vi "DAC Run.vi"(8 "error in":errorcluster, 11 "DAC CS Humid in":refnum<class "DAC CS Humid.lvclass">) -> (0 "error out":errorcluster, 3 "DAC CS Humid out":refnum<class "DAC CS Humid.lvclass">)   [LabVIEW 2019, in "DAC.lvlib" / "DAC CS Humid.lvclass"]
uses:
  DAC CS Humid.lvclass
  C:/Users/wg/Documents/LV_Projects/test-stand/App/DAC/DAC.lvclass
  DAC.lvclass/DAC.ctl
  Results/Results Method.ctl
  Results/DeepU Results/DeepU Results.lvclass
  DAC CS Humid.lvclass/DAC CS Humid.ctl
  <vilib>/DAQmx/miscellaneous.llb/DAQmx Fill In Error Info.vi
  DAC.lvclass
  Results/Results.lvlib
  <vilib>/DAQmx/read.llb/DAQmx Read (Analog 1D Wfm NChan 1Samp).vi
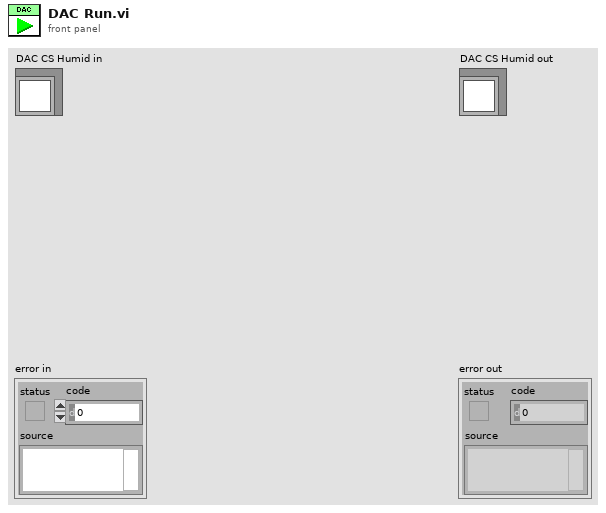
[diagram p1: front panel]
types:
  T1 = typedef "Results.lvlib/Results Method.ctl" = enum16{"Get", "Set"}
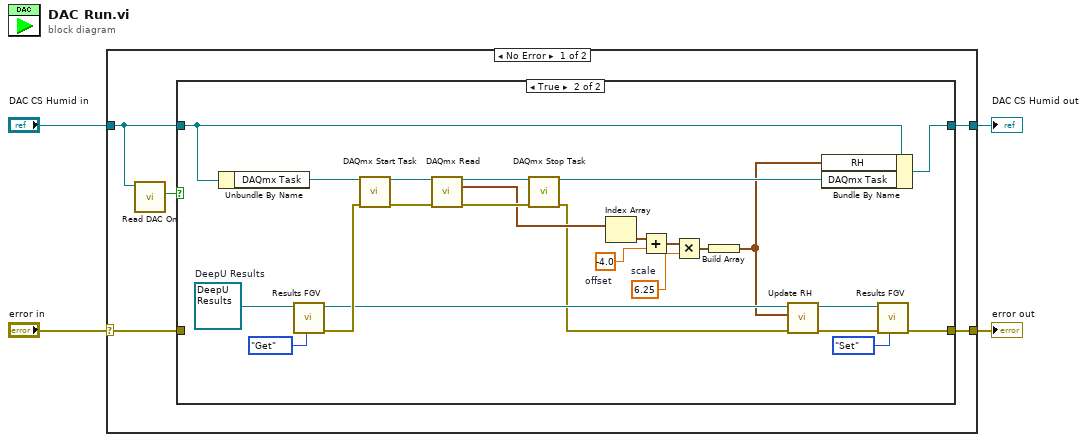
[diagram p0: block diagram]
diagram:
  n1 = case shown="No Error" "error in" {
    selector: "error in" -> [w7 w37]
    tunnel: [w6 w37] -> w2
    tunnel: [w8 w36] -> w1
    tunnel: "DAC CS Humid in" -> [w5 w36]
    frame No Error {
      n2 = call "Read DAC On.vi"("DAC in"=w5) -> ("DAC On"=w9:bool)  [unwired: 8 in, 2 out]
      n3 = case shown="True" w9 {
        tunnel: w5 -> [w11 w30]
        tunnel: [w11 w29] -> w8
        tunnel: w7 -> [w10 _]
        tunnel: [w10 w24] -> w6
        frame False {
        }
        frame True {
          w14 = 6.25  # scale
          w16 = -4.0  # offset
          w27 = refnum<class "DeepU Results.lvclass"> refnum  # DeepU Results
          n4 = Unbundle By Name(w30) -> ("DAQmx Task"=w35:refnum<k21>)
          n5 = call-dynamic "Results FGV.vi"("Method"=Results_Method."Get", "DeepU Results in"=w27) -> ("error out"=w23:errorcluster, "DeepU Results out"=w21:refnum<class "DeepU Results.lvclass">)  [unwired: 8 in]
          n6 = call <vilib>:"DAQmx Start Task.vi"("task/channels in"=w35, "error in"=w23) -> ("task out"=w34:refnum<k21>, "error out"=w32:errorcluster)  [unwired: 12 in]
          n7 = call-poly <vilib>:"DAQmx Read.vi"("task/channels in"=w34, "error in"=w32) -> ("task out"=w33:refnum<k21>, "data"=w19:waveform(dbl)[], "error out"=w31:errorcluster)  [unwired: 11 in]
          n8 = call <vilib>:"DAQmx Stop Task.vi"("task/channels in"=w33, "error in"=w31) -> ("task out"=w28:refnum<k21>, "error out"=w12:errorcluster)  [unwired: 12 in]
          n9 = Index Array(array=w19) -> (element=w17:waveform(dbl))  [unwired: 1 in]
          n10 = Add(x=w17, y=w16) -> (x+y=w15:waveform(dbl))
          n11 = Multiply(x=w15, y=w14) -> (x*y=w13:waveform(dbl))
          n12 = Build Array(w13) -> (w18:waveform(dbl)[])
          n13 = call "Update RH.vi"("error in"=w12, "RH"=w18, "DeepU Results in"=w21) -> ("error out"=w22:errorcluster, "DeepU Results out"=w20:refnum<class "DeepU Results.lvclass">)  [unwired: 7 in]
          n14 = Bundle By Name(cluster=w30, "RH"=w18, "DAQmx Task"=w28) -> (w29:refnum<class "DAC CS Humid.lvclass">)
          n15 = call-dynamic "Results FGV.vi"("Method"=Results_Method."Set", "error in"=w22, "DeepU Results in"=w20) -> ("error out"=w24:errorcluster)  [unwired: 7 in, 1 out]
        }
      }
    }
    frame Error {
    }
  }
  "error out" <- w2
  "DAC CS Humid out" <- w1
